vi "Xbox One Controller to Joystick State.vi"(9 "Joystick State In":cluster{"Buttons":T1[], "Axis":T2[]}, 10 "Xbox One Controller":T3 {"Right Joystick"."Right" min=-1.0 max=1.0 step=0.1 scale=-1.0..1.0; "Right Joystick"."Forward" min=-1.0 max=1.0 step=0.1 scale=-1.0..1.0; "Left Joystick"."Right" min=-1.0 max=1.0 step=0.1 scale=-1.0..1.0; "Left Joystick"."Forward" min=-1.0 max=1.0 step=0.1 scale=-1.0..1.0}) -> (2 "Joystick State Out":cluster{"Buttons":T1[], "Axis":T2[]})   [LabVIEW 2014, in "Xbox One Controller.lvlib"]
uses:
  Xbox One Controller.lvlib
  Xbox One Controller State.ctl
  Joystick.ctl
  Joystick/Joystick Class/Button State.ctl
  Joystick/Joystick Class/Axis State.ctl
  Joystick/Joystick Class/Joystick.lvclass
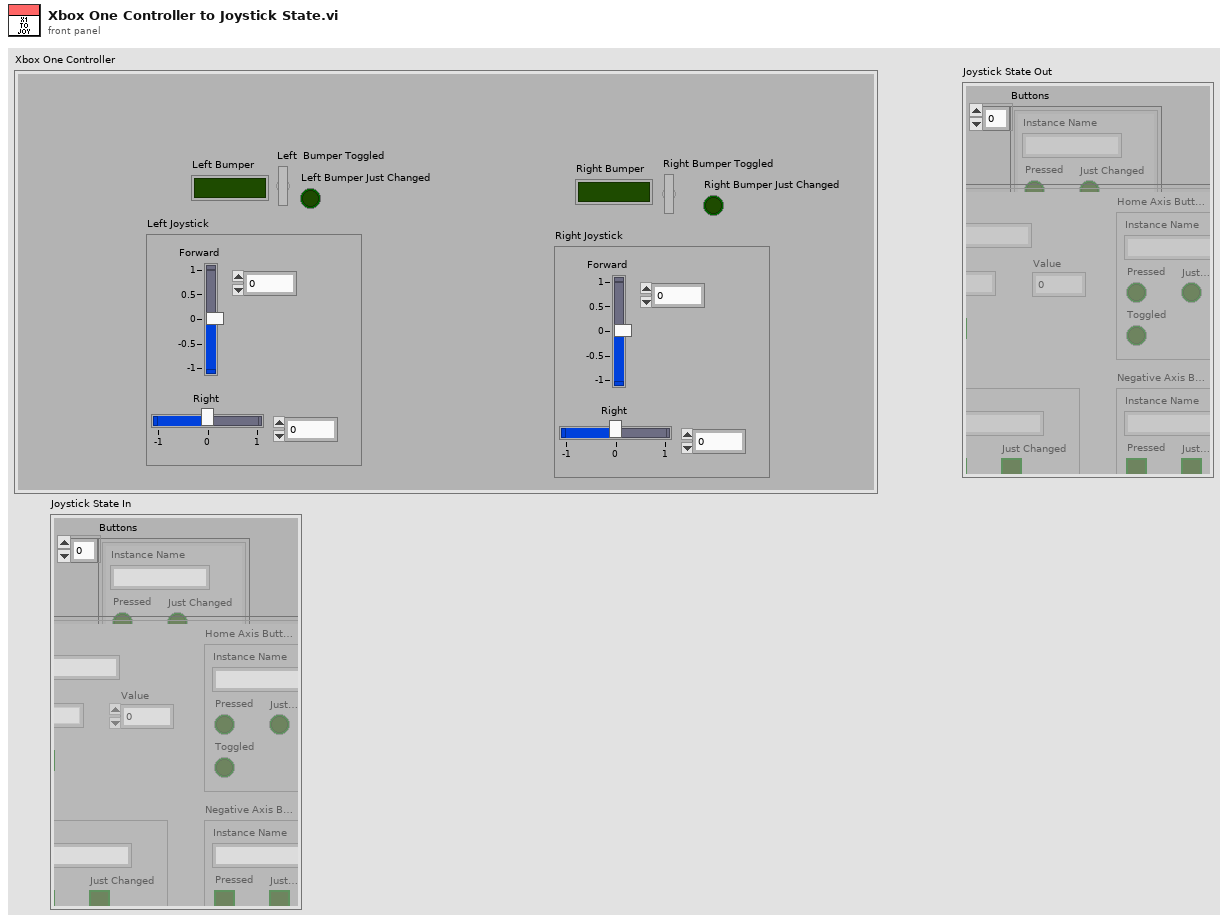
[diagram p1: front panel]
types:
  T1 = typedef "Joystick.lvlib/Joystick.lvclass/Button State.ctl" = cluster{"Pressed":bool, "Instance Name":string, "Toggled":bool, "Just Changed":bool}
  T2 = typedef "Joystick.lvlib/Joystick.lvclass/Axis State.ctl" = cluster{"Instance Name":string, "Deadband":dbl, "Value":dbl, "At Home":bool, "Postive Axis Button State":T1, "Negative Axis Button State":T1, "Home Axis Button State":T1}
  T3 = typedef "Xbox One Controller.lvlib/Xbox One Controller State.ctl" = cluster{"Left Joystick":T4, "Right Joystick":T4, "Right Bumper":bool, "Left Bumper":bool, "Left  Bumper Toggled":bool, "Right Bumper Toggled":bool, "Left Bumper Just Changed":bool, "Right Bumper Just Changed":bool}
  T4 = typedef "Xbox One Controller.lvlib/Joystick.ctl" = cluster{"Forward":dbl, "Right":dbl}
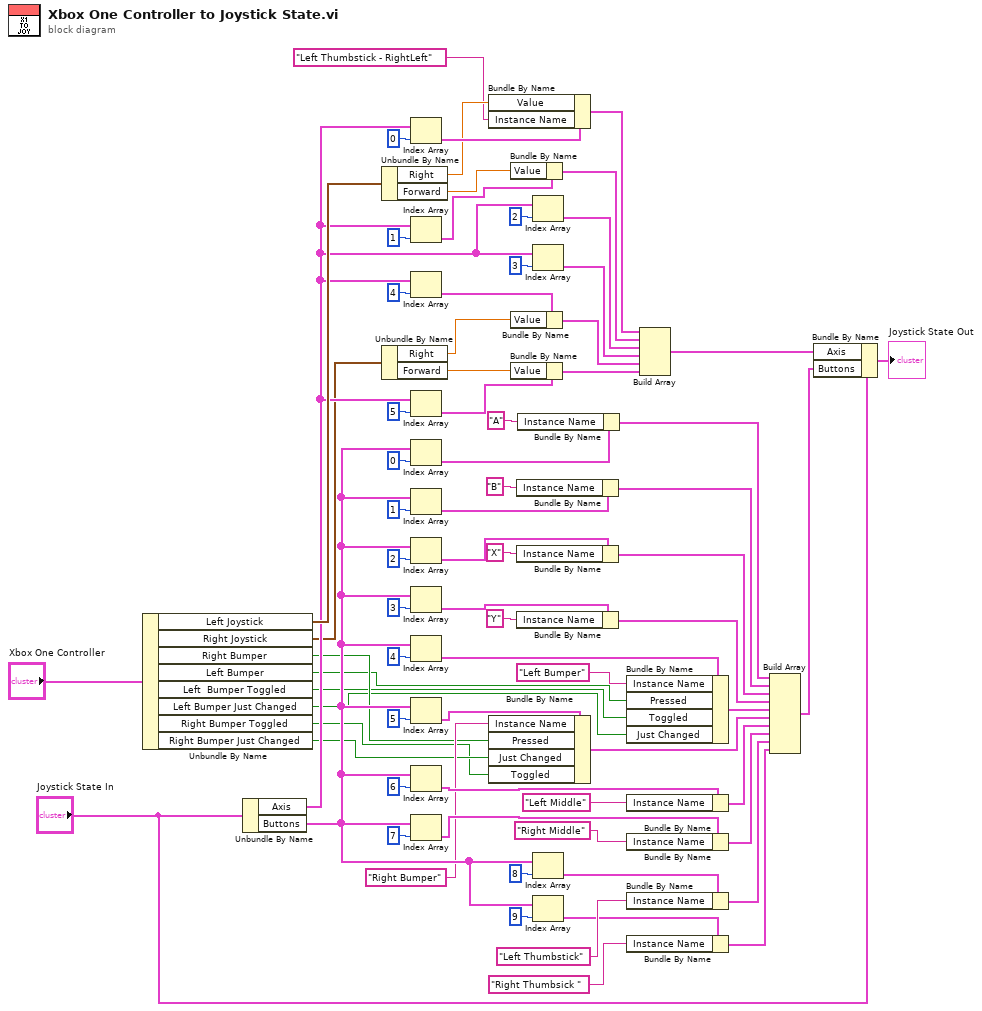
[diagram p0: block diagram]
diagram:
  n1 = Unbundle By Name("Xbox One Controller") -> ("Left Joystick"=w71:T4, "Right Joystick"=w57:T4, "Right Bumper"=w6:bool, "Left Bumper"=w5:bool, "Left  Bumper Toggled"=w4:bool, "Left Bumper Just Changed"=w3:bool, "Right Bumper Toggled"=w1:bool, "Right Bumper Just Changed"=w2:bool)
  n2 = Unbundle By Name("Joystick State In") -> ("Axis"=w60:T2[], "Buttons"=w38:T1[])
  n3 = Unbundle By Name(w71) -> ("Right"=w70:dbl, "Forward"=w67:dbl)
  n4 = Unbundle By Name(w57) -> ("Right"=w55:dbl, "Forward"=w53:dbl)
  n5 = Index Array(array=w60, index=0) -> (element=w72:T2)
  n6 = Index Array(array=w60, index=1) -> (element=w68:T2)
  n7 = Index Array(array=w60, index=4) -> (element=w56:T2)
  n8 = Index Array(array=w60, index=5) -> (element=w54:T2)
  n9 = Index Array(array=w38, index=0) -> (element=w39:T1)
  n10 = Index Array(array=w38, index=1) -> (element=w33:T1)
  n11 = Index Array(array=w38, index=2) -> (element=w30:T1)
  n12 = Index Array(array=w38, index=3) -> (element=w28:T1)
  n13 = Index Array(array=w38, index=4) -> (element=w27:T1)
  n14 = Index Array(array=w38, index=5) -> (element=w26:T1)
  n15 = Index Array(array=w38, index=6) -> (element=w25:T1)
  n16 = Index Array(array=w38, index=7) -> (element=w24:T1)
  n17 = Bundle By Name(cluster=w72, "Value"=w70, "Instance Name"="Left Thumbstick - RightLeft") -> (w66:T2)
  n18 = Bundle By Name(cluster=w26, "Instance Name"="Right Bumper", "Pressed"=w6, "Just Changed"=w2, "Toggled"=w1) -> (w16:T1)
  n19 = Bundle By Name(cluster=w68, "Value"=w67) -> (w65:T2)
  n20 = Bundle By Name(cluster=w56, "Value"=w55) -> (w52:T2)
  n21 = Bundle By Name(cluster=w54, "Value"=w53) -> (w51:T2)
  n22 = Bundle By Name(cluster=w33, "Instance Name"="B") -> (w32:T1)
  n23 = Bundle By Name(cluster=w30, "Instance Name"="X") -> (w29:T1)
  n24 = Bundle By Name(cluster=w28, "Instance Name"="Y") -> (w10:T1)
  n25 = Bundle By Name(cluster=w39, "Instance Name"="A") -> (w35:T1)
  n26 = Index Array(array=w60, index=2) -> (element=w59:T2)
  n27 = Index Array(array=w60, index=3) -> (element=w58:T2)
  n28 = Index Array(array=w38, index=8) -> (element=w13:T1)
  n29 = Index Array(array=w38, index=9) -> (element=w9:T1)
  n30 = Bundle By Name(cluster=w27, "Instance Name"="Left Bumper", "Pressed"=w5, "Toggled"=w4, "Just Changed"=w3) -> (w17:T1)
  n31 = Bundle By Name(cluster=w25, "Instance Name"="Left Middle") -> (w15:T1)
  n32 = Bundle By Name(cluster=w24, "Instance Name"="Right Middle") -> (w14:T1)
  n33 = Bundle By Name(cluster=w13, "Instance Name"="Left Thumbstick") -> (w11:T1)
  n34 = Bundle By Name(cluster=w9, "Instance Name"="Right Thumbsick ") -> (w7:T1)
  n35 = Build Array(w66, w65, w59, w58, w52, w51) -> (w50:T2[])
  n36 = Build Array(w35, w32, w29, w10, w17, w16, w15, w14, w11, w7) -> (w36:T1[])
  n37 = Bundle By Name(cluster="Joystick State In", "Axis"=w50, "Buttons"=w36) -> (→"Joystick State Out":cluster{"Buttons":T1[], "Axis":T2[]})
